vi "Delete Icon Editor from LV Installation.vi"(8 "error in":errorcluster) -> (0 "error out":errorcluster, 3 "were files previously present?":bool)   [LabVIEW 2021]
uses:
  <vilib>/Utility/error.llb/Error Cluster From Error Code.vi
  <vilib>/ErrorRing/Error Ring.xnode
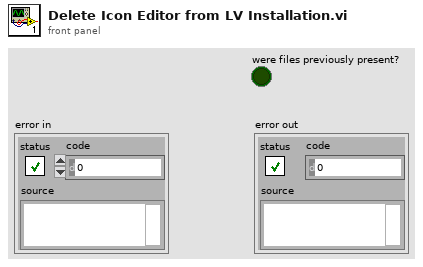
[diagram p1: front panel]
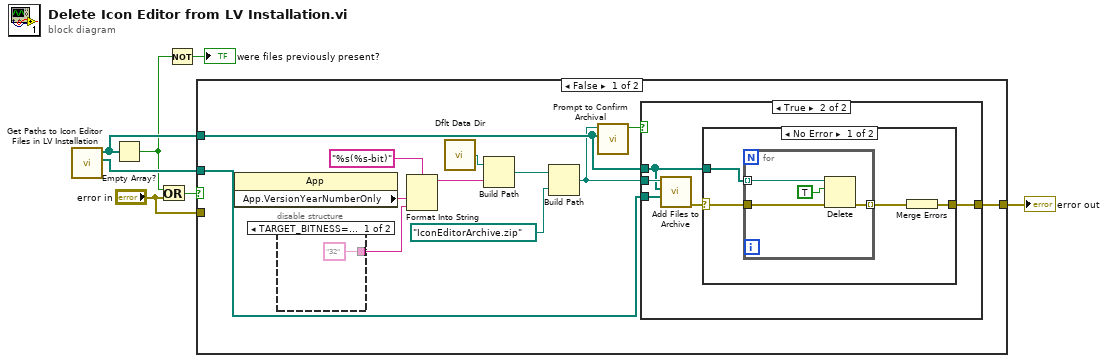
[diagram p0: block diagram]
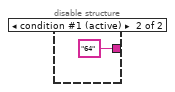
[diagram p2: hidden frame]
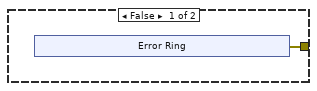
[diagram p3: hidden frame]
diagram:
  n1 = call "Get Paths to Icon Editor Files in LV Installation.vi"() -> ("relative paths"=w4:path[], "absolute paths"=w3:path[])  [unwired: 10 in]
  n2 = Empty Array?(array=w3) -> (empty?=w1:bool)
  n3 = Or(x=w1, y="error in") -> (x .or. y?=w5:bool)
  n4 = Not(x=w1) -> (.not. x?=→"were files previously present?":bool)
  n5 = case shown="False" w5 {
    tunnel: w3 -> [w18 _]
    tunnel: w4 -> [w9 _]
    tunnel: "error in" -> [_ w41]
    tunnel: [w8 w41] -> w7
    frame False {
      n6 = property class="App"() -> ("App.VersionYearNumberOnly"=w15:string)  [unwired: 2 in, 2 out]
      n7 = disable-structure shown="TARGET_BITNESS==32" {
        disable-tunnel: ["32" "64"] -> w16
        frame condition #0 {
        }
        frame condition #1 (active) {
        }
      }
      n8 = Format Into String(format string="%s(%s-bit)", w15, w16) -> (resulting string=w13:string)  [unwired: 2 in, 1 out]
      n9 = call <vilib>:"Dflt Data Dir.vi"() -> ("App:Default Data Directory"=w14:path)
      n10 = Build Path(base path=w14, name or relative path=w13) -> (appended path=w12:path)
      n11 = Build Path(base path=w12, name or relative path=path "IconEditorArchive.zip") -> (appended path=w10:path)
      n12 = call "Prompt to Confirm Archival.vi"("files to be deleted"=w18, "archive destination"=w10) -> ("confirmed?"=w19:bool)  [unwired: 9 in]
      n13 = case shown="True" w19 {
        tunnel: w18 -> [_ w29]
        tunnel: w10 -> [_ w31]
        tunnel: w9 -> [_ w30]
        tunnel: [w22 w27] -> w8
        frame False {
          n14 = xnode "Error Ring"() -> ("error out"=w22:errorcluster)
        }
        frame True {
          n15 = call "Add Files to Archive.vi"("relative paths in zip"=w30, "absolute source paths"=w29, "zip path"=w31) -> ("error out"=w28:errorcluster)  [unwired: 8 in]
          n16 = case shown="No Error" w28 {
            selector: w28 -> [w34 w40]
            tunnel: w29 -> [w35 _]
            tunnel: [w32 w40] -> w27
            frame No Error {
              n17 = for {
                tunnel: w35 -> [w38] mode=indexing
                tunnel: w34 -> [w37]
                tunnel: [w36] -> w33 mode=indexing
                n18 = Delete(path (use dialog)=w38, entire hierarchy (F)=TRUE, error in=w37) -> (error out=w36:errorcluster)  [unwired: 2 in, 2 out]
              }
              n19 = Merge Errors(w33) -> (w32:errorcluster)
            }
            frame Error {
            }
          }
        }
      }
    }
    frame True {
    }
  }
  "error out" <- w7
